vi "A33LoadArbitraryVolat_py.vi"() -> ()   [LabVIEW 2022 SP3]
doc: "Creates and saves an arbitrary waveform in edit memory. \n\n<B>Note:</B>\n\nCreates an arbitrary waveform in edit memory and because of this, the waveform will remain stored on the instrument until deleted. If any sensitive information is contained in the arbitrary waveform, it is recommended that the waveform be deleted when finished."
panel:
  in  "Array WFM 2":i16[](array[numeric])
  in  "WFM Source 2":u16(ring) items=["Single file", "Split files", "Array"]
  in  "ARB Number 2":u32=1
  in  "Channel (1: Channel1) 2":u16(ring)=1 items=["Channel1"=1, "Channel2"=2]
  in  "Timeout (40000 ms) 2":u32=40000
  in  "WFM Length 2":i32
  in  "WFM (Column) Number 2":i32
  in  "WFM Path 2":path
  # "Load waveform into arb\nmemory of a certain channel\nunder name 'ARB#'\nIf WFM alerady exists - use ClearArbitrary\n64M points in total per channel\nTimeout is not implemented, because this\nVI is inline-compatible, need external timeout\nincrease"
  # "No dots in the file name!"
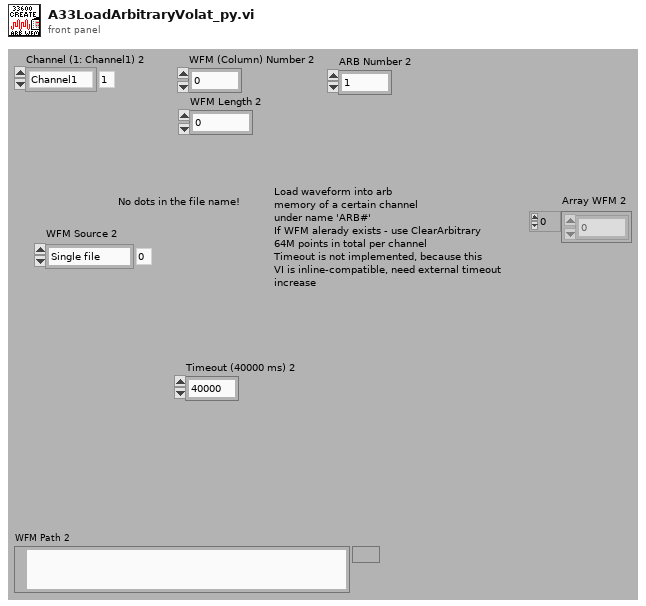
[diagram p1: front panel]
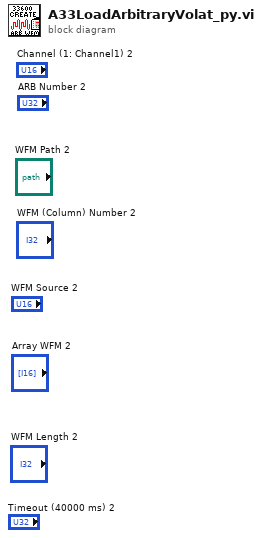
[diagram p0: block diagram]
diagram:
